vi "SWERVE_TRAJECTORY_UPDATE_DIAG_INFO.vi"(8 "AtReference":bool, 9 "OutputTRAJ_STATE":T1 {"POSE"."ROTATION"."SIN" format="%13.4f"; "POSE"."ROTATION"."COS" format="%13.4f"; "POSE"."ROTATION"."VALUE" format="%13.4f"; "POSE"."TRANSLATION"."Y" format="%14.3f"; "POSE"."TRANSLATION"."X" format="%14.3f"}, 10 "Error and Corr":T5 {"Error Pose"."ROTATION"."SIN" format="%13.4f"; "Error Pose"."ROTATION"."COS" format="%13.4f"; "Error Pose"."ROTATION"."VALUE" format="%13.4f"; "Error Pose"."TRANSLATION"."Y" format="%14.3f"; "Error Pose"."TRANSLATION"."X" format="%14.3f"}, 11 "Orientation Target":dbl) -> ()   [LabVIEW 2019]
uses:
  <vilib>/Rock Robotics/WPI/ThirdParty/JAS_Junk/TrajLib/Trajectory_Library.lvlib
  SWERVE_TRAJECTORY_GLOBALS.vi
  <vilib>/Rock Robotics/WPI/ThirdParty/JAS_Junk/TrajLib/TypeDef/TRANSLATION2D.ctl
  <vilib>/Rock Robotics/WPI/ThirdParty/JAS_Junk/TrajLib/TypeDef/ROTATION2D.ctl
  <vilib>/Rock Robotics/WPI/ThirdParty/JAS_Junk/TrajLib/TypeDef/POSE2D.ctl
  <vilib>/Rock Robotics/WPI/ThirdParty/JAS_Junk/TrajLib/TypeDef/TRAJ_STATE.ctl
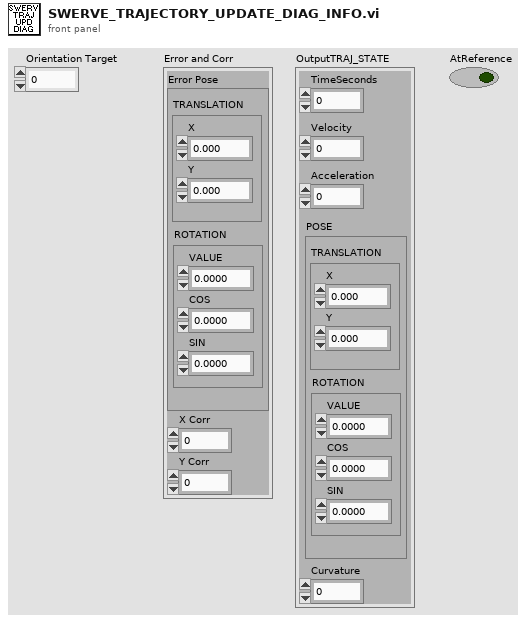
[diagram p1: front panel]
types:
  T1 = typedef "Trajectory_Library.lvlib/TRAJ_STATE.ctl" = cluster{"TimeSeconds":dbl, "Velocity":dbl, "Acceleration":dbl, "POSE":T2, "Curvature":dbl}
  T2 = typedef "Trajectory_Library.lvlib/POSE2D.ctl" = cluster{"TRANSLATION":T3, "ROTATION":T4}
  T3 = typedef "Trajectory_Library.lvlib/TRANSLATION2D.ctl" = cluster{"X":dbl, "Y":dbl}
  T4 = typedef "Trajectory_Library.lvlib/ROTATION2D.ctl" = cluster{"VALUE":dbl, "COS":dbl, "SIN":dbl}
  T5 = cluster{"Error Pose":T2, "X Corr":dbl, "Y Corr":dbl}
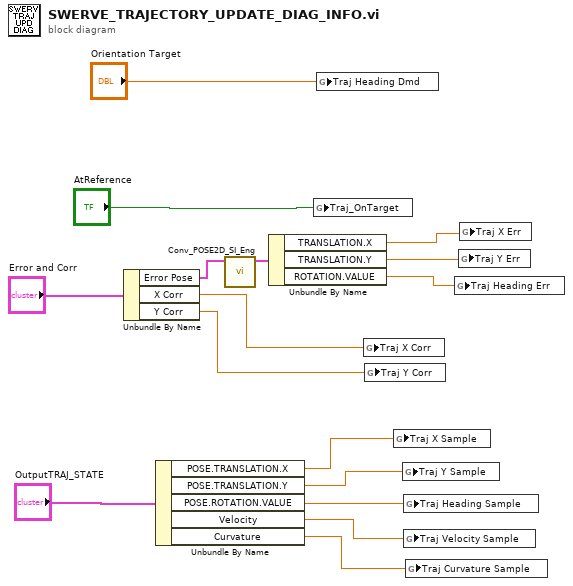
[diagram p0: block diagram]
diagram:
  n1 = Unbundle By Name("Error and Corr") -> ("Error Pose"=w16:T2, "X Corr"=w6:dbl, "Y Corr"=w7:dbl)
  n2 = Unbundle By Name("OutputTRAJ_STATE") -> ("POSE.TRANSLATION.X"=w12:dbl, "POSE.TRANSLATION.Y"=w11:dbl, "POSE.ROTATION.VALUE"=w10:dbl, "Velocity"=w9:dbl, "Curvature"=w8:dbl)
  n3 = call <vilib>:"Conv_POSE2D_SI_Eng.vi"("Err Pose in SI"=w16) -> ("Err Pose out ENG"=w13:T2)  [unwired: 10 in]
  n4 = Unbundle By Name(w13) -> ("TRANSLATION.X"=w5:dbl, "TRANSLATION.Y"=w4:dbl, "ROTATION.VALUE"=w3:dbl)
  n5 = global write "SWERVE_TRAJECTORY_GLOBALS.vi" "Traj_OnTarget"("AtReference") -> ()
  n6 = global write "SWERVE_TRAJECTORY_GLOBALS.vi" "Traj Heading Dmd"("Orientation Target") -> ()
  n7 = global write "SWERVE_TRAJECTORY_GLOBALS.vi" "Traj X Corr"(w6) -> ()
  n8 = global write "SWERVE_TRAJECTORY_GLOBALS.vi" "Traj Y Corr"(w7) -> ()
  n9 = global write "SWERVE_TRAJECTORY_GLOBALS.vi" "Traj X Sample"(w12) -> ()
  n10 = global write "SWERVE_TRAJECTORY_GLOBALS.vi" "Traj Y Sample"(w11) -> ()
  n11 = global write "SWERVE_TRAJECTORY_GLOBALS.vi" "Traj Heading Sample"(w10) -> ()
  n12 = global write "SWERVE_TRAJECTORY_GLOBALS.vi" "Traj Velocity Sample"(w9) -> ()
  n13 = global write "SWERVE_TRAJECTORY_GLOBALS.vi" "Traj Curvature Sample"(w8) -> ()
  n14 = global write "SWERVE_TRAJECTORY_GLOBALS.vi" "Traj Heading Err"(w3) -> ()
  n15 = global write "SWERVE_TRAJECTORY_GLOBALS.vi" "Traj Y Err"(w4) -> ()
  n16 = global write "SWERVE_TRAJECTORY_GLOBALS.vi" "Traj X Err"(w5) -> ()
